vi "Write Stream Fields.vi"(8 "error in (no error)":errorcluster, 10 "Stream Fields":string[](array[string]), 11 "LokiJsonFormatter in":refnum<class "LokiJsonFormatter.lvclass">) -> (0 "error out":errorcluster, 3 "LokiJsonFormatter out":refnum<class "LokiJsonFormatter.lvclass">)   [LabVIEW 2019, in "hse-logger.lvlib" / "LokiJsonFormatter.lvclass"]
uses:
  LokiJsonFormatter.lvclass
  LokiJsonFormatter.lvclass/LokiJsonFormatter.ctl
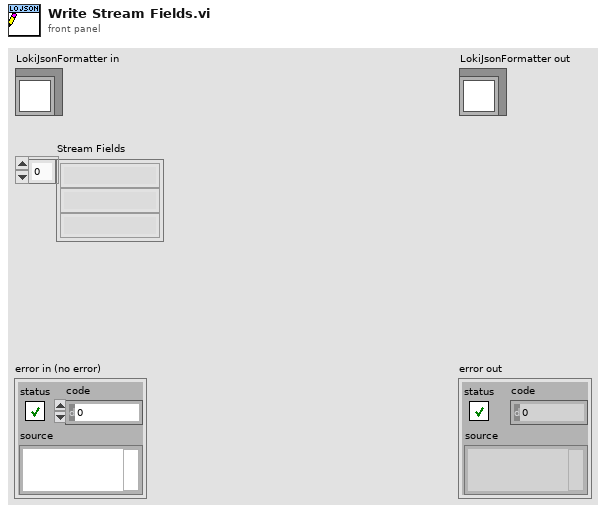
[diagram p1: front panel]
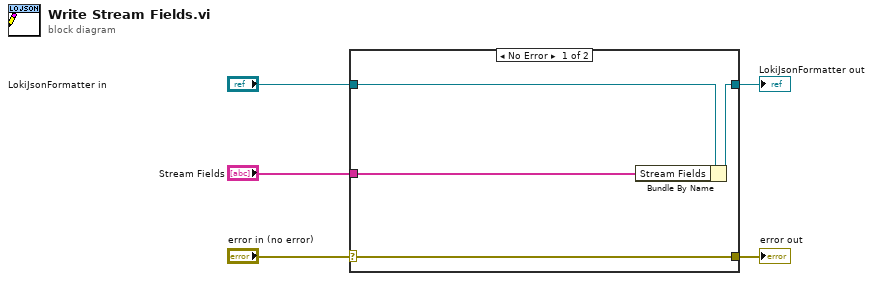
[diagram p0: block diagram]
diagram:
  n1 = case shown="No Error" "error in (no error)" {
    selector: "error in (no error)" -> [w9 w10]
    tunnel: [w9 w10] -> w4
    tunnel: [w7 w11] -> w2
    tunnel: "LokiJsonFormatter in" -> [w8 w11]
    tunnel: "Stream Fields" -> [w6 _]
    frame No Error {
      n2 = Bundle By Name(cluster=w8, "Stream Fields"=w6) -> (w7:refnum<class "LokiJsonFormatter.lvclass">)
    }
    frame Error {
    }
  }
  "error out" <- w4
  "LokiJsonFormatter out" <- w2
